vi "http write header.vi"(8 "error in (no error)":errorcluster, 10 "application request":T1, 11 "TCP Network Connection in":refnum<k5>) -> (0 "error out":errorcluster, 3 "TCP Network Connection out":refnum<k5>)   [LabVIEW 2013]
uses:
  http response.ctl
  http response packet type.ctl
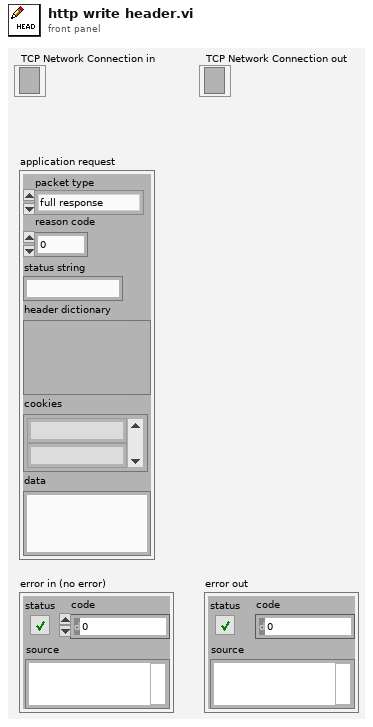
[diagram p1: front panel]
types:
  T1 = typedef "http response.ctl" = cluster{"packet type":T2, "reason code":u16, "status string":string, "header dictionary":variant, "cookies":string[], "data":string}
  T2 = typedef "http response packet type.ctl" = enum16{"full response", "header only", "data only", "last data"}
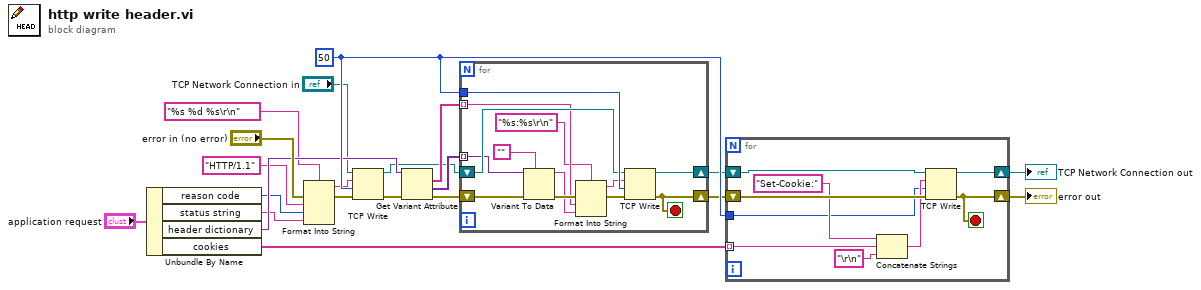
[diagram p0: block diagram]
diagram:
  w20 = 50 ("timeout ms (25000)")
  n1 = Unbundle By Name("application request") -> ("reason code"=w4:u16, "status string"=w3:string, "header dictionary"=w10:variant, "cookies"=w17:string[])
  n2 = Format Into String(format string="%s %d %s\r\n", error in="error in (no error)", "HTTP/1.1" ("input 1"), w4, w3) -> (resulting string=w7:string, error out=w8:errorcluster)  [unwired: 1 in]
  n3 = TCP Write(connection ID="TCP Network Connection in", data in=w7, error in (no error)=w8, 9:w20) -> (connection ID out=w9:refnum<k5>, error out=w12:errorcluster)  [unwired: 1 out]
  n4 = Get Variant Attribute(Variant=w10, error in=w12) -> (names=w14:string[], values=w13:variant[], error out=w11:errorcluster)  [unwired: 2 in, 1 out]
  n5 = for {
    shift-right: [w34] -> w15
    shift-left: w9 -> [w32]
    shift-right: [w22] -> w16
    shift-left: w11 -> [w31]
    tunnel: w20 -> [w33]
    tunnel: w13 -> [w29] mode=indexing
    tunnel: w14 -> [w26] mode=indexing
    stop <- w22 stop-if-true
    n6 = Variant To Data(error in=w31, type="", Variant=w29) -> (data=w25:string, error out=w30:errorcluster)
    n7 = Format Into String(format string="%s:%s\r\n", error in=w30, w26, w25) -> (resulting string=w23:string, error out=w27:errorcluster)  [unwired: 1 in]
    n8 = TCP Write(connection ID=w32, data in=w23, error in (no error)=w27, 9:w33) -> (connection ID out=w34:refnum<k5>, error out=w22:errorcluster)  [unwired: 1 out]
  }
  n9 = for {
    shift-right: [w43] -> w18
    shift-left: w15 -> [w42]
    shift-right: [w40] -> w19
    shift-left: w16 -> [w41]
    tunnel: w17 -> [w37] mode=indexing
    tunnel: w20 -> [w35]
    stop <- w40 stop-if-true
    n10 = Concatenate Strings("Set-Cookie:" ("string"), w37, "\r\n" ("format string")) -> (w36:string)
    n11 = TCP Write(connection ID=w42, data in=w36, error in (no error)=w41, 9:w35) -> (connection ID out=w43:refnum<k5>, error out=w40:errorcluster)  [unwired: 1 out]
  }
  "error out" <- w19
  "TCP Network Connection out" <- w18
